vi "set task token if null.vi"(10 "task token":refnum<class "null task token.lvclass">, 11 "task in":refnum<class "task.lvclass">) -> (3 "task out":refnum<class "task.lvclass">)   [LabVIEW 2013, in "task.lvclass"]
uses:
  task.lvclass
  task token/null task token.lvclass
  task.lvclass/task.ctl
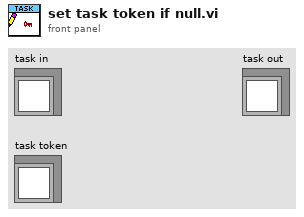
[diagram p1: front panel]
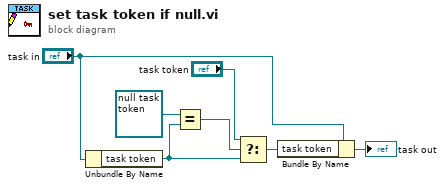
[diagram p0: block diagram]
diagram:
  n1 = Unbundle By Name("task in") -> ("task token"=w3:refnum<class "null task token.lvclass">)
  n2 = Equal?(x=refnum<class "null task token.lvclass"> refnum ("null task token"), y=w3) -> (x = y?=w4:bool)
  n3 = Select(t="task token", s=w4, f=w3) -> (s? t:f=w1:refnum<class "null task token.lvclass">)
  n4 = Bundle By Name(cluster="task in", "task token"=w1) -> (→"task out":refnum<class "task.lvclass">)
